vi "根据规格存OKNG图存数据到缓存.vi"(6 "错误常量":errorcluster caption="错误in", 7 "结果":bool, 8 "选择相机字符串":string="相机1", 9 "存档数据和结果":T1, 10 "当前零件型号":string="771自动锁螺丝", 11 "Img输入":T2) -> ()   [LabVIEW 2014]
uses:
  <vilib>/vision/Image Controls.llb/IMAQ Image.ctl
  Global.vi
  SaveTestDataSubVI/SaveTestDataAction.ctl
  <vilib>/Utility/file.llb/Write To Spreadsheet File (DBL).vi
panel:
  out "添加的路径":path
  out "当天存数据路径":path
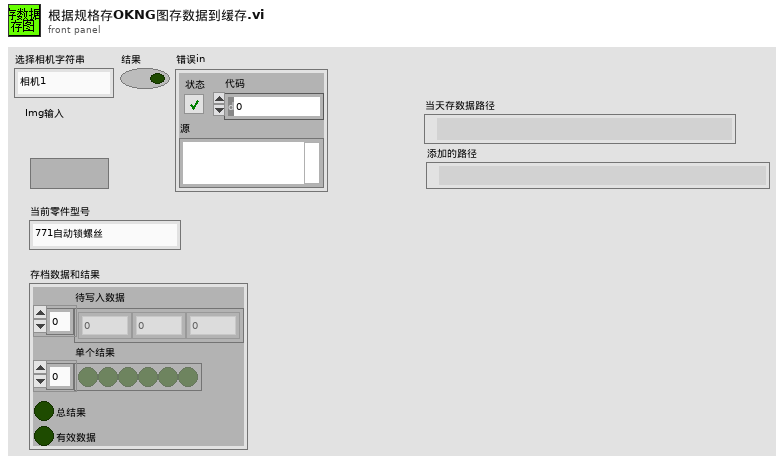
[diagram p1: front panel]
types:
  T1 = typedef "控件-存档数据和结果.ctl" = cluster{"待写入数据":dbl[], "单个结果":bool[], "总结果":bool, "有效数据":bool}
  T2 = typedef "IMAQ Image.ctl" = refnum<image>
  T3 = typedef "OtherSpec.ctl" = cluster{"其它勾选类规格":T4, "其它数据类规格":T5, "相机名称":T6, "参数":cluster{"Mark1曝光时间":i32, "Mark2曝光时间":i32, "二维码曝光时间":i32}}
  T4 = typedef "其它勾选类规格.ctl" = cluster{"保存图片":bool, "上传设备状态数据":bool, "保存数据":bool, "开机默认开启监控摄像头":bool, "启用mark拍照 ":bool}
  T5 = typedef "其他数据类规格.ctl" = cluster{"相机1像素-毫米换算系数":dbl, "相机2像素-毫米换算系数":dbl, "D盘剩余空间预警(G)":dbl, "视频最长录制时间(秒)":dbl}
  T6 = typedef "相机名称品牌使用状态.ctl" = cluster{"相机1名称":T7, "相机2名称":T7, "Cam1启用":bool, "Cam2启用":bool, "Basler1":bool, "Basler2":bool}
  T7 = typedef "IMAQdx.ctl" = refnum<k21>
  T8 = typedef "SaveTestDataAction.ctl" = enum16{"初始化", "更新机种规格", "读取表格", "第N次拍照数据写入表格(缓存)", "Mark点拍照数据存档", "取料拍螺帽数据存档", "复锁拍螺帽数据存档", "关闭表格", "打开表格"}
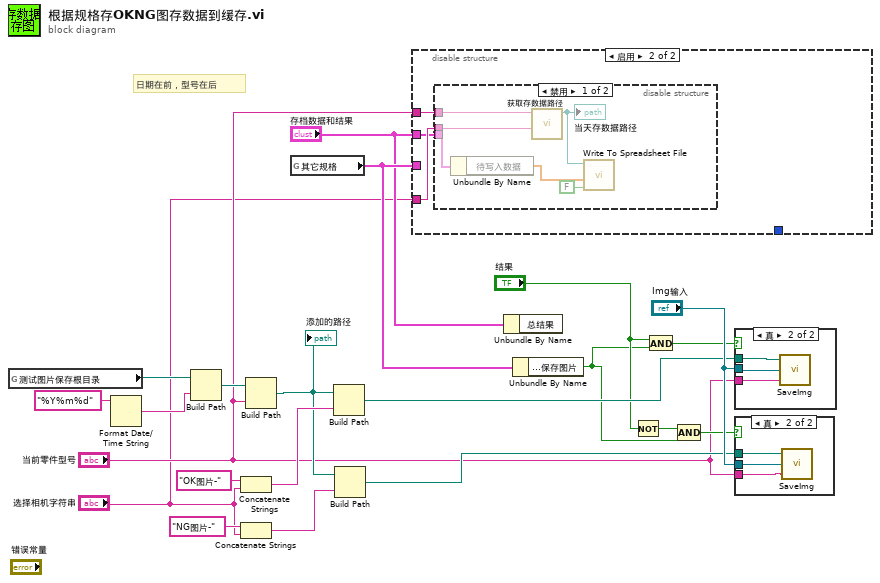
[diagram p0: block diagram]
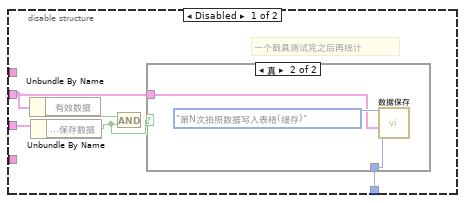
[diagram p2: hidden frame]
diagram:
  # "日期在前，型号在后"
  n1 = global read "Global.vi" "测试图片保存根目录"() -> (w15:path)
  n2 = Format Date/Time String(time format string (%c)="%Y%m%d") -> (date/time string=w8:string)  [unwired: 2 in]
  n3 = Build Path(base path=w15, name or relative path=w8) -> (appended path=w7:path)
  n4 = Concatenate Strings("OK图片-" ("字符串"), "选择相机字符串") -> (w13:string)
  n5 = Concatenate Strings("NG图片-" ("字符串"), "选择相机字符串") -> (w10:string)
  n6 = Build Path(base path=w7, name or relative path="当前零件型号") -> (appended path=w6:path)
  "添加的路径" <- w6
  n7 = global read "Global.vi" "其它规格"() -> (w20:T3)
  n8 = Build Path(base path=w6, name or relative path=w13) -> (appended path=w5:path)
  n9 = Build Path(base path=w6, name or relative path=w10) -> (appended path=w11:path)
  n10 = disable-structure shown="启用" {
    disable-tunnel: w20 -> [w25 _]
    disable-tunnel: "存档数据和结果" -> [w24 w30]
    disable-tunnel: _ -> [w22 _]
    disable-tunnel: "当前零件型号" -> [_ w32]
    disable-tunnel: "选择相机字符串" -> [_ w31]
    frame Disabled {
      # "一个载具测试完之后再统计"
      n11 = Unbundle By Name(w24) -> ("有效数据"=w26:bool)
      n12 = Unbundle By Name(w25) -> ("其它勾选类规格.保存数据"=w23:bool)
      n13 = And(x=w26, y=w23) -> ()  [unwired: 1 out]
      n14 = case shown="真" w23 {
        tunnel: w24 -> [_ w28]
        tunnel: w22 -> [_ w27]
        frame False {
        }
        frame True {
          n15 = call "数据保存.vi"("单个产品拍照点序号(1开始)"=w27, "存档数据和结果"=w28, "选项"=SaveTestDataAction."第N次拍照数据写入表格(缓存)") -> ()  [unwired: 5 in, 2 out]
        }
      }
    }
    frame Enabled {
      n16 = disable-structure shown="禁用" {
        disable-tunnel: w32 -> [w38 _]
        disable-tunnel: w31 -> [w37 _]
        disable-tunnel: w30 -> [w36 _]
        frame Disabled {
          n17 = Unbundle By Name(w36) -> ("待写入数据"=w35:dbl[])
          n18 = call "获取存数据路径.vi"(9:w37, "ModelEditInfo"=w38) -> ("当天存数据路径"=w34:path)  [unwired: 9 in]
          "当天存数据路径" <- w34
          n19 = call-poly <vilib>:"Write To Spreadsheet File.vi"("append to file? (new file:F)"=FALSE, "1D data"=w35, "file path (dialog if empty)"=w34) -> ()  [unwired: 5 in, 1 out]
        }
        frame Enabled {
        }
      }
    }
  }
  n20 = Unbundle By Name("存档数据和结果") -> ()  [unwired: 1 out]
  n21 = Unbundle By Name(w20) -> ("其它勾选类规格.保存图片"=w1:bool)
  n22 = Not(x="结果") -> (.not. x?=w18:bool)
  n23 = And(x="结果", y=w1) -> (x .and. y?=w19:bool)
  n24 = Compound Arithmetic op=AND(w18, w1) -> (w17:bool)
  n25 = case shown="真" w19 {
    tunnel: w5 -> [_ w41]
    tunnel: "Img输入" -> [_ w40]
    tunnel: "当前零件型号" -> [_ w39]
    frame False {
    }
    frame True {
      n26 = call "SaveImg.vi"("零件型号"=w39, "Image"=w40, "Fold路径"=w41) -> ()
    }
  }
  n27 = case shown="真" w17 {
    tunnel: "Img输入" -> [_ w44]
    tunnel: w11 -> [_ w43]
    tunnel: "当前零件型号" -> [_ w42]
    frame False {
    }
    frame True {
      n28 = call "SaveImg.vi"("零件型号"=w42, "Image"=w44, "Fold路径"=w43) -> ()
    }
  }
